vi "rqcAlice ServiceNET Send Command.vi"(8 "error in":errorcluster, 10 "command":T1, 11 "rqcAlice ServiceNET in":T2) -> (0 "error out":errorcluster, 3 "rqcAlice ServiceNET out":T2)   [LabVIEW 2019]
uses:
  Custom Controls/rqcAlice ServiceNET control.ctl
  Custom Controls/rqc ServiceNET command.ctl
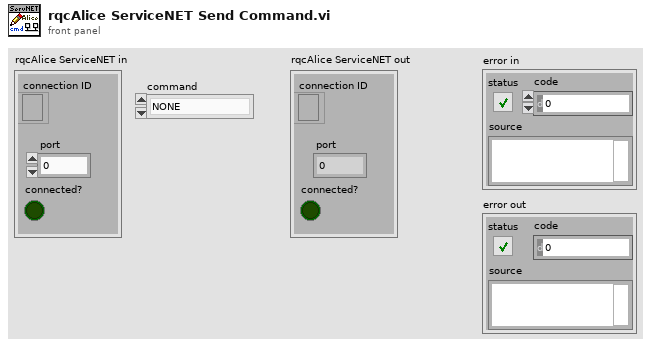
[diagram p1: front panel]
types:
  T1 = typedef "rqc ServiceNET command.ctl" = enum8{"NONE", "READY", "START", "PING"}
  T2 = typedef "rqcAlice ServiceNET control.ctl" = cluster{"connection ID":refnum<k5>, "port":u16, "connected?":bool}
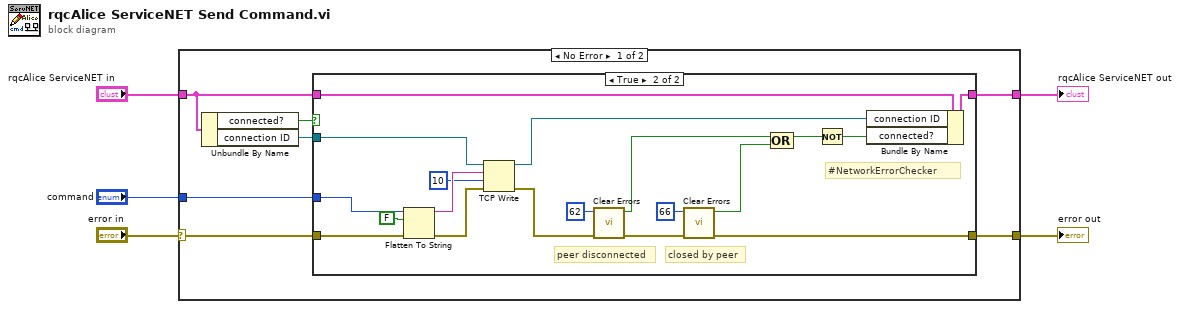
[diagram p0: block diagram]
diagram:
  n1 = case shown="No Error" "error in" {
    selector: "error in" -> [w8 w35]
    tunnel: [w7 w35] -> w4
    tunnel: "rqcAlice ServiceNET in" -> [w11 w34]
    tunnel: [w10 w34] -> w2
    tunnel: "command" -> [w6 _]
    frame No Error {
      n2 = Unbundle By Name(w11) -> ("connected?"=w12:bool, "connection ID"=w9:refnum<k5>)
      n3 = case shown="True" w12 {
        tunnel: [w14 w32] -> w10
        tunnel: w11 -> [w14 w33]
        tunnel: w9 -> [_ w29]
        tunnel: w8 -> [w13 w27]
        tunnel: [w13 w18] -> w7
        tunnel: w6 -> [_ w26]
        frame False {
        }
        frame True {
          # "closed by peer"
          # "peer disconnected"
          # "#NetworkErrorChecker"
          n4 = Flatten To String(anything=w26, prepend array or string size? (T)=FALSE, error in (no error)=w27) -> (data string=w24:string, error out=w25:errorcluster)  [unwired: 1 in, 1 out]
          n5 = TCP Write(connection ID=w29, data in=w24, error in (no error)=w25, 9:10 ("timeout ms (25000)")) -> (connection ID out=w23:refnum<k5>, error out=w22:errorcluster)  [unwired: 1 out]
          n6 = call <vilib>:"Clear Errors.vi"("error in (no error)"=w22, "specific error code to clear (0: all)"=62) -> ("error out"=w19:errorcluster, "specific error cleared?"=w30:bool)  [unwired: 4 in]
          n7 = call <vilib>:"Clear Errors.vi"("error in (no error)"=w19, "specific error code to clear (0: all)"=66) -> ("error out"=w18:errorcluster, "specific error cleared?"=w15:bool)  [unwired: 4 in]
          n8 = Compound Arithmetic op=OR(w30, w15) -> (w16:bool)
          n9 = Not(x=w16) -> (.not. x?=w31:bool)
          n10 = Bundle By Name(cluster=w33, "connection ID"=w23, "connected?"=w31) -> (w32:T2)
        }
      }
    }
    frame Error {
    }
  }
  "rqcAlice ServiceNET out" <- w2
  "error out" <- w4
